vi "PH_PSDBController.destructor.vi"(0 "i ref in":refnum<vi>, 5 "error in(no error)":errorcluster) -> (19 "error out":errorcluster)   [LabVIEW 2014, in "PH_PSDBController.lvlib"]
doc: "This is the destructor of a class.\n\nLicense Agreement for this software:\n\nCopyright (C)\nGesellschaft für Schwerionenforschung, GSI\nPlanckstr. 1\n64291 Darmstadt\nGermany\n\nContact: D.Beck@gsi.de \n\nThis program is free software; you can redistribute it and/or modify it under the terms of the \nGNU General Public License as published by the Free Software Foundation; either version 2 of \nthe license, or (at your option) any later version.\n\nThis program is distributed in the hope that it will be useful, but WITHOUT ANY WARRANTY; \nwithout even the implied warranty of MERCHANTABILITY or FITNESS FOR A PARTICULAR PURPOSE. See the GNU General License for more details (http://www.gnu.org).\n\nGesellschaft für Schwerionenforschung, GSI\nPlanckstr. 1, 64291 Darmstadt, Germany\nFor all questions and ideas contact: M.Richter@gsi.de, H.Brand@gsi.de or D.Beck@gsi.de.\nLast update: 16-JUN-2004"
uses:
  PH_PSDBController.lvlib
  lib.lib/DimLVEvent/LVDimInterface/LVDimInterface.lvlib
  PH_StatusHandler/PH_StatusHandler.lvlib
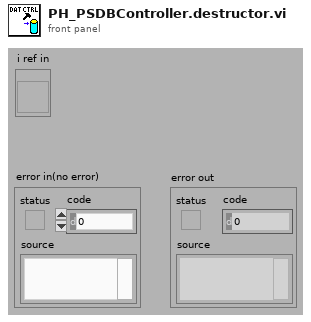
[diagram p1: front panel]
types:
  T1 = typedef "PH_PSDBController.lvlib/PH_PSDBController.i attribute.ctl" = cluster{"GUI Refs":cluster{"Data Status":refnum<vi>, "Current Shot ID":refnum<vi>, "active Subsystems":refnum<vi>, "Experiment Description":refnum<vi>, "Shot Comment":refnum<vi>, "Experiment":refnum<vi>, "Shottype":refnum<vi>, "Sequencer SM State":refnum<vi>, "Instances with Errors":refnum<vi>}, "Service ID Shot ID":i32, "Service ID wanted Subsystem":i32, "Data Status":T2, "Shotinformation":cluster{"Current Experiment ID":i32, "Current Shot Type":i32, "Current Comment":string}, "Data taking?":bool, "Service ID current Shottype":i32, "Service ID current Experiment":i32, "Service ID currentShot Comment":i32, "Service ID possible Shottypes":i32, "Service ID possible Experiments":i32, "possible Experiments":T3[], "possible Shottypes":T3[], "List":cluster{"Info":cluster{"Instance":string, "Data Status":T2}[], "GUI Ref":refnum<vi>, "Classname":string}[], "Subsystems Off?":cluster{"PHELIX_Beamline_fs_YLF_BL_Status":bool, "PHELIX_Beamline_ns_BL_Status":bool, "PHELIX_Beamline_PA_Input_BL_Status":bool, "PHELIX_Beamline_PA_MA_BL_Status":bool, "PHELIX_Beamline_MA_Z6_BL_Status":bool, "PHELIX_Beamline_MA_LB_BL_Status":bool, "PHELIX_Beamline_PA_LL_BL_Status":bool}, "PSDB Credentials":T4}
  T2 = typedef "PH_PSDBWriter.lvlib/PH_PSDBWriter.Data Status.ctl" = i16
  T3 = typedef "PSDB.lvlib/PSDB_Info.ctl" = cluster{"Name":string, "Description":string, "ID":i32}
  T4 = typedef "PH_Common.lvlib/PH_Connection.PSDB Credentials.ctl" = cluster{"PW":string, "ID":string, "DS":string}
  T5 = enum16{"SetAttribute", "GetAttribute", "CreateAttribute", "DestroyAttribute", "DestroyAllAtributes"}
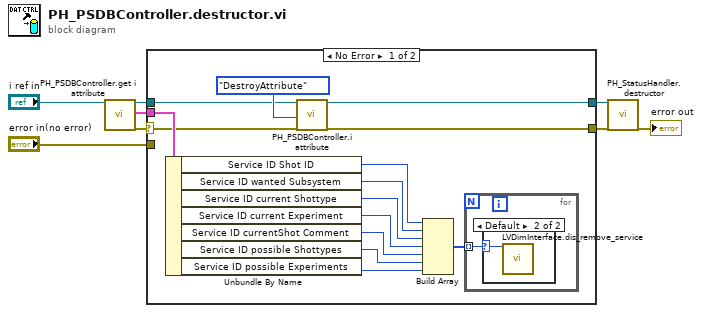
[diagram p0: block diagram]
diagram:
  n1 = call "PH_PSDBController.get i attribute.vi"("i ref in"="i ref in") -> ("i ref out"=w6:refnum<vi>, "i attribute"=w5:T1, "error out"=w2:errorcluster)  [unwired: 16 in]
  n2 = case shown="No Error" w2 {
    selector: w2 -> [w9 _]
    tunnel: [w21 w25] -> w8
    tunnel: w6 -> [w20 w25]
    tunnel: w5 -> [w18 _]
    tunnel: [w10 w26] -> w4
    tunnel: "error in(no error)" -> [_ w26]
    frame No Error {
      n3 = Unbundle By Name(w18) -> ("Service ID Shot ID"=w17:i32, "Service ID wanted Subsystem"=w13:i32, "Service ID current Shottype"=w16:i32, "Service ID current Experiment"=w15:i32, "Service ID currentShot Comment"=w14:i32, "Service ID possible Shottypes"=w12:i32, "Service ID possible Experiments"=w11:i32)
      n4 = call "PH_PSDBController.i attribute.vi"("VI Refnum"=w20, "Action"=T5."DestroyAttribute", "error in (no error)"=w9) -> ("VI Refnum out"=w21:refnum<vi>, "error out"=w10:errorcluster)  [unwired: 14 in, 1 out]
      n5 = Build Array(w17, w13, w16, w15, w14, w12, w11) -> (w19:i32[])
      n6 = for {
        tunnel: w19 -> [w23] mode=indexing
        n7 = case shown="Default" w23 {
          selector: w23 -> [_ w24]
          frame -1 {
          }
          frame Default {
            n8 = call "LVDimInterface.dis_remove_service.vi"("my_serviceID"=w24) -> ()  [unwired: 18 in, 1 out]
          }
        }
      }
    }
    frame Error {
    }
  }
  n9 = call "PH_StatusHandler.destructor.vi"("i ref in"=w8, "error in(no error)"=w4) -> ("error out"=→"error out":errorcluster)  [unwired: 17 in]
